vi "Data Server Encode Response Filename.vi"(6 "Command ID":T1, 8 "error in (no error)":errorcluster, 10 "Filename":string, 11 "Time Stamp":timestamp) -> (0 "error out":errorcluster, 3 "Output string":string)   [LabVIEW 2011, in "Data Server VIs.lvlib"]
uses:
  Data Server VIs.lvlib
  Types Definitions/Type Data Server Command ID.ctl
  Type Definitions.lvlib
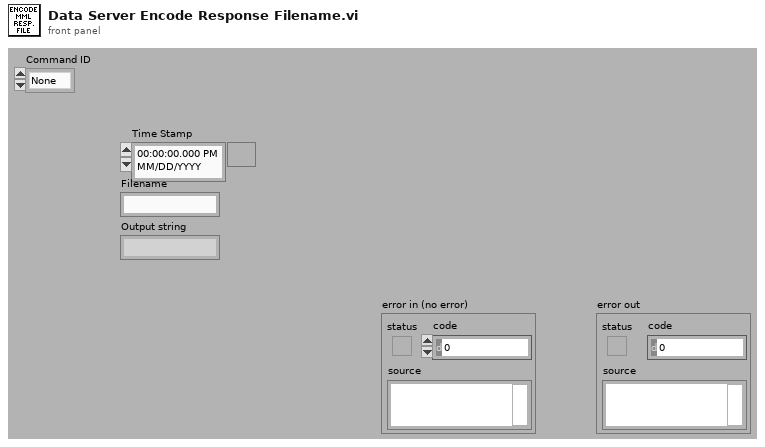
[diagram p1: front panel]
types:
  T1 = typedef "Type Definitions.lvlib/Type Data Server Command ID.ctl" = enum16{"None", "FA_Start", "FA_Stop", "Update_Controller"}
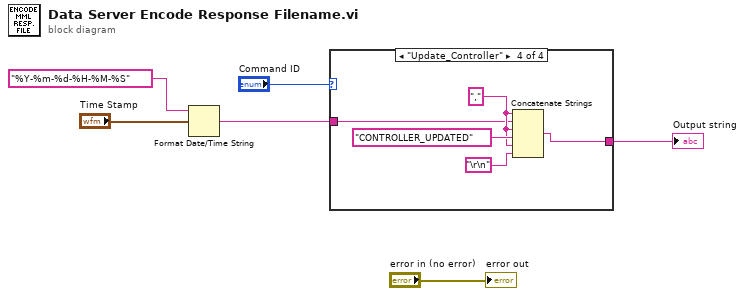
[diagram p0: block diagram]
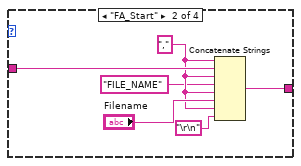
[diagram p3: hidden frame]
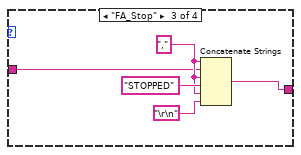
[diagram p4: hidden frame]
diagram:
  n1 = Format Date/Time String(time format string (%c)="%Y-%m-%d-%H-%M-%S", seconds (now)="Time Stamp") -> (date/time string=w4:string)  [unwired: 1 in]
  n2 = case shown="\"Update_Controller\"" "Command ID" {
    tunnel: w4 -> [_ w12 w14 w19]
    tunnel: [_ w8 w13 w18] -> w3
    frame "None", Default {
    }
    frame "FA_Start" {
      w10 = "," ("string")
      n3 = Concatenate Strings(w10, w12, w10, "FILE_NAME" ("string"), w10, "Filename", w10, "\r\n") -> (w8:string)
    }
    frame "FA_Stop" {
      w15 = "," ("string")
      n4 = Concatenate Strings(w15, w14, w15, "STOPPED" ("string"), w15, "\r\n") -> (w13:string)
    }
    frame "Update_Controller" {
      w20 = "," ("string")
      n5 = Concatenate Strings(w20, w19, w20, "CONTROLLER_UPDATED" ("string"), w20, "\r\n") -> (w18:string)
    }
  }
  "Output string" <- w3
  "error out" <- "error in (no error)"
